vi "Pre-Dig User Hook.vi"(8 "Error In":errorcluster) -> (0 "Error Out":errorcluster)   [LabVIEW 2018, in "Tests.lvlib" / "Toolkit.lvlib" / "Integration.lvlib"]
uses:
  Integration.lvlib
  Support/Hook Search Paths.ctl
  src/Toolkit/Toolkit.lvlib
  <vilib>/addons/_JKI Toolkits/Caraya/classes/Test/Test.lvclass
  Tests.lvlib
  <vilib>/addons/_JKI Toolkits/Caraya/classes/Assert/Assert.lvclass
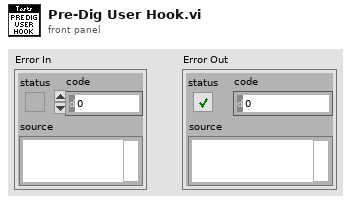
[diagram p1: front panel]
types:
  T1 = typedef "Tests.lvlib/Toolkit.lvlib/Integration.lvlib/Hook Search Paths.ctl" = enum32{"System", "User", "Project (Hidden)", "Project (Visible)"}
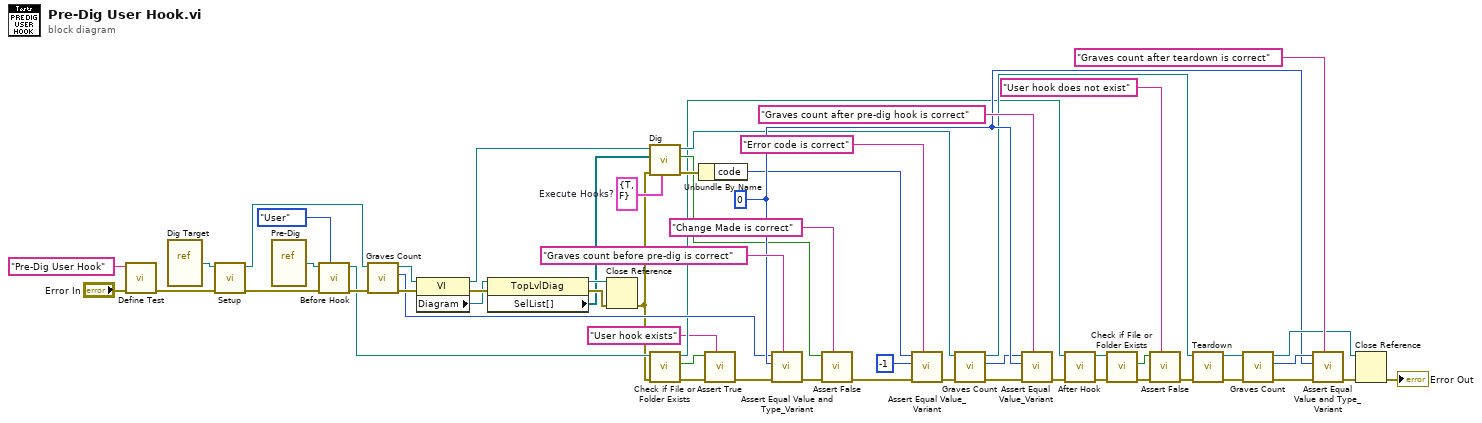
[diagram p0: block diagram]
diagram:
  w38 = cluster{"Pre":bool, "Post":bool} {"Pre"=TRUE, "Post"=FALSE}  # Execute Hooks?
  w43 = 0 ("size(s)")
  n1 = call <vilib>:"Define Test.vi"("error in (no error)"="Error In", "Label (VI Title)"="Pre-Dig User Hook") -> ("error out"=w53:errorcluster)  [unwired: 9 in]
  n2 = vi-ref "Dig Target.vi"() -> (w39:refnum<vi>)
  n3 = call "Setup.vi"("Error In"=w53, "VI In"=w39) -> ("Error Out"=w28:errorcluster, "VI Out"=w17:refnum<vi>)  [unwired: 8 in]
  n4 = vi-ref "Pre-Dig.vi"() -> (w29:refnum<vi>)
  n5 = call "Before Hook.vi"("Hooks Search Path"=Hook_Search_Paths."User", "Error In"=w28, "Hook VI"=w29) -> ("Error Out"=w18:errorcluster, "Hook VI"=w12:path)  [unwired: 7 in]
  n6 = call "Graves Count.vi"("Error In"=w18, "Test Target In"=w17) -> ("Error Out"=w24:errorcluster, "Graves Count"=w14:i32, "Test Target Out"=w23:refnum<vi>)  [unwired: 7 in]
  n7 = property class="VI"(reference=w23, error in=w24) -> (reference out=w16:refnum<vi>, error out=w20:errorcluster, "Diagram"=w19:refnum<vi>)
  n8 = property class="TopLvlDiag"(reference=w19, error in=w20) -> (reference out=w22:refnum<vi>, error out=w21:errorcluster, "SelList[]"=w15:refnum<vi>[])
  n9 = Close Reference(reference=w22, error in (no error)=w21) -> (error out=w8:errorcluster)
  n10 = call "Dig.vi"("Execute Hooks?"=w38, "Error In"=w8, "Selection List"=w15, "VI In"=w16) -> ("Error Out"=w42:errorcluster, "Change Made?"=w31:bool, "VI Out"=w35:refnum<vi>)  [unwired: 5 in]
  n11 = call <vilib>:"Check if File or Folder Exists.vi"("error in (no error)"=w8, "path"=w12) -> ("error out"=w13:errorcluster, "file or folder exists?"=w10:bool, "dup path"=w11:path)  [unwired: 7 in]
  n12 = Unbundle By Name(w42) -> ("code"=w41:i32)
  n13 = call <vilib>:"Assert True.vi"("Label"="User hook exists", "error in (no error)"=w13, "True?"=w10) -> ("error out"=w9:errorcluster)  [unwired: 8 in]
  n14 = call <vilib>:"Assert Equal Value and Type_Variant.vi"("Label"="Graves count before pre-dig is correct", "error in (no error)"=w9, "Y"=w43, "X"=w14) -> ("error out"=w52:errorcluster)  [unwired: 7 in]
  n15 = call <vilib>:"Assert False.vi"("Label"="Change Made is correct", "error in (no error)"=w52, "False?"=w31) -> ("error out"=w32:errorcluster)  [unwired: 8 in]
  n16 = call <vilib>:"Assert Equal Value_Variant.vi"("Label"="Error code is correct", "error in (no error)"=w32, "Y"=-1 ("code"), "X"=w41) -> ("error out"=w37:errorcluster)  [unwired: 7 in]
  n17 = call "Graves Count.vi"("Error In"=w37, "Test Target In"=w35) -> ("Error Out"=w36:errorcluster, "Graves Count"=w33:i32, "Test Target Out"=w34:refnum<vi>)  [unwired: 7 in]
  n18 = call <vilib>:"Assert Equal Value_Variant.vi"("Label"="Graves count after pre-dig hook is correct", "error in (no error)"=w36, "Y"=w43, "X"=w33) -> ("error out"=w26:errorcluster)  [unwired: 7 in]
  n19 = call "After Hook.vi"("Error In"=w26, "Hook VI In"=w11) -> ("Error Out"=w4:errorcluster, "Hook VI Out"=w5:path)  [unwired: 8 in]
  n20 = call <vilib>:"Check if File or Folder Exists.vi"("error in (no error)"=w4, "path"=w5) -> ("error out"=w3:errorcluster, "file or folder exists?"=w6:bool)  [unwired: 7 in, 1 out]
  n21 = call <vilib>:"Assert False.vi"("Label"="User hook does not exist", "error in (no error)"=w3, "False?"=w6) -> ("error out"=w2:errorcluster)  [unwired: 8 in]
  n22 = call "Teardown.vi"("Error In"=w2, "VI In"=w34) -> ("Error Out"=w46:errorcluster, "VI Out"=w48:refnum<vi>)  [unwired: 8 in]
  n23 = call "Graves Count.vi"("Error In"=w46, "Test Target In"=w48) -> ("Error Out"=w45:errorcluster, "Graves Count"=w44:i32, "Test Target Out"=w47:refnum<vi>)  [unwired: 7 in]
  n24 = call <vilib>:"Assert Equal Value and Type_Variant.vi"("Label"="Graves count after teardown is correct", "error in (no error)"=w45, "Y"=w43, "X"=w44) -> ("error out"=w50:errorcluster)  [unwired: 7 in]
  n25 = Close Reference(reference=w47, error in (no error)=w50) -> (error out=→"Error Out":errorcluster)
